vi "Get Src-Sink Terminal by Name.vi"(9 "Poosible Terminal Names":string[](array[string]), 10 "Find Source":bool=TRUE, 11 "Event Case Termianls":refnum<vi>[](array[refnum])) -> (3 "Term Refnum out":refnum<vi>)   [LabVIEW 2019, in "gRPC Template Creation Utility.lvlib"]
uses:
  gRPC Template Creation Utility.lvlib
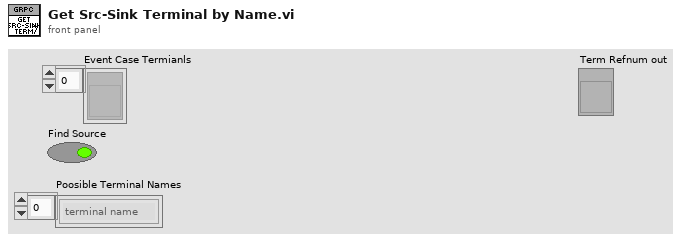
[diagram p1: front panel]
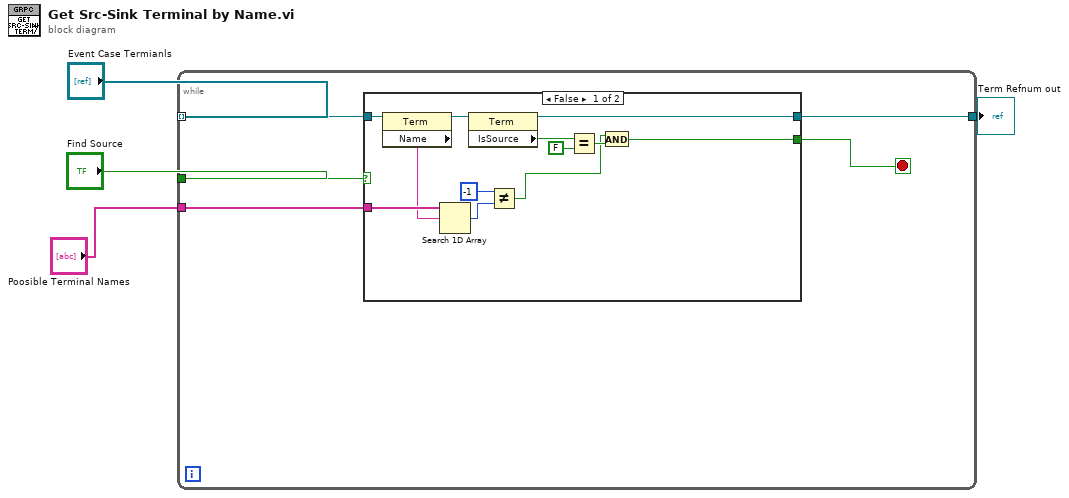
[diagram p0: block diagram]
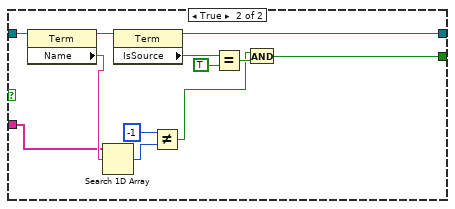
[diagram p2: hidden frame]
diagram:
  n1 = while {
    tunnel: "Event Case Termianls" -> [w9] mode=indexing
    tunnel: "Find Source" -> [w8]
    tunnel: [w6] -> w2
    tunnel: "Poosible Terminal Names" -> [w5]
    stop <- w7 stop-if-true
    n2 = case shown="False" w8 {
      tunnel: w9 -> [w21 w33]
      tunnel: [w17 w29] -> w7
      tunnel: [w15 w28] -> w6
      tunnel: w5 -> [w14 w22]
      frame False {
        n3 = property class="Term"(reference=w21) -> (reference out=w16:refnum<vi>, "Name"=w13:string)  [unwired: 1 in, 1 out]
        n4 = Search 1D Array(1D array=w14, element=w13) -> (index of element=w12:i32)  [unwired: 1 in]
        n5 = property class="Term"(reference=w16) -> (reference out=w15:refnum<vi>, "IsSource"=w20:bool)  [unwired: 1 in, 1 out]
        n6 = Not Equal?(x=-1, y=w12) -> (x != y?=w10:bool)
        n7 = Equal?(x=w20, y=FALSE) -> (x = y?=w18:bool)
        n8 = And(x=w10, y=w18) -> (x .and. y?=w17:bool)
      }
      frame True {
        n9 = property class="Term"(reference=w33) -> (reference out=w32:refnum<vi>, "Name"=w23:string)  [unwired: 1 in, 1 out]
        n10 = Search 1D Array(1D array=w22, element=w23) -> (index of element=w26:i32)  [unwired: 1 in]
        n11 = property class="Term"(reference=w32) -> (reference out=w28:refnum<vi>, "IsSource"=w31:bool)  [unwired: 1 in, 1 out]
        n12 = Not Equal?(x=-1, y=w26) -> (x != y?=w24:bool)
        n13 = Equal?(x=w31, y=TRUE) -> (x = y?=w27:bool)
        n14 = And(x=w24, y=w27) -> (x .and. y?=w29:bool)
      }
    }
  }
  "Term Refnum out" <- w2
